vi "IP Address - DHCP.vi"(11 "error in (no error)":errorcluster) -> (4 "return code":i32, 6 "standard output":string, 8 "standard error":string, 15 "error out":errorcluster)   [LabVIEW 2009]
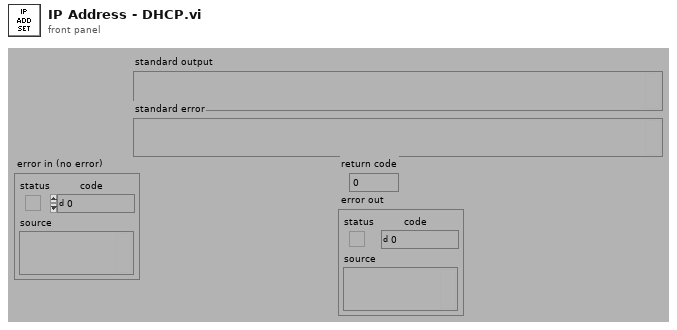
[diagram p1: front panel]
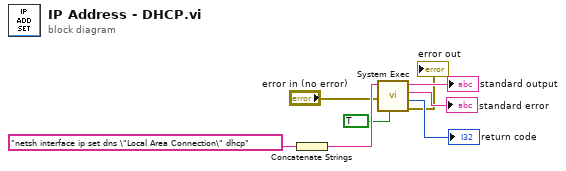
[diagram p0: block diagram]
diagram:
  n1 = Concatenate Strings("netsh interface ip set dns \"Local Area Connection\" dhcp" ("command line")) -> (w8:string)
  n2 = call <vilib>:"System Exec.vi"("run minimized? (F)"=TRUE, "error in (no error)"="error in (no error)", "command line"=w8) -> ("error out"=→"error out":errorcluster, "return code"=→"return code":i32, "standard error"=→"standard error":string, "standard output"=→"standard output":string)  [unwired: 5 in]
